vi "String value arrange_0.vi"() -> ()   [LabVIEW 2015]
panel:
  in  "Tab Control":enum32{"Page 1"}(tab)
  out "String mixx":string="100,101,102,103,104,105,106,107,108,109"
  out "Totall String charter":i32
  out "string addres":i32[](array[numeric])
  out "correct string":string[](array[string])
  out "Totall String":i16
  out "after substring":string
  out "before substring":string
  # "String value arrange"
  # "Pardeep Kumar"
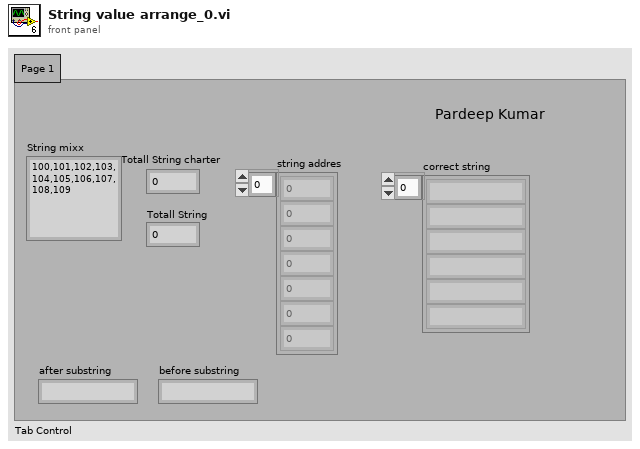
[diagram p1: front panel]
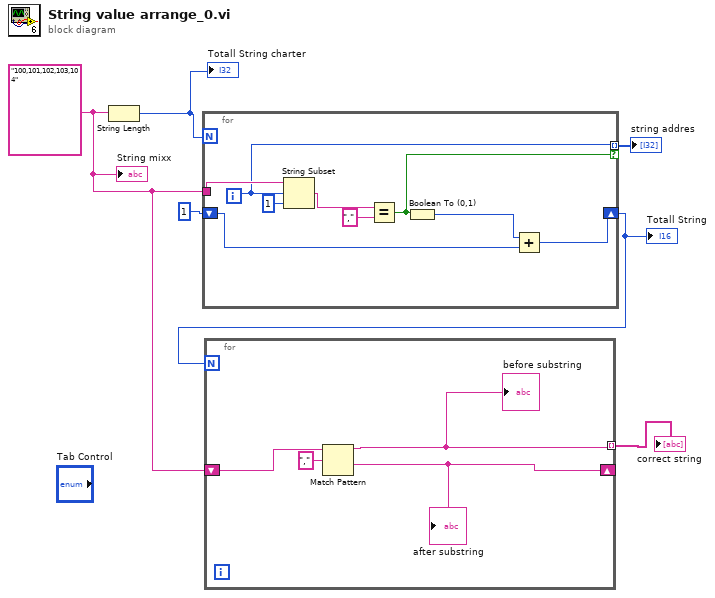
[diagram p0: block diagram]
diagram:
  w3 = "100,101,102,103,104"
  n1 = String Length(string=w3) -> (length=w6:i32)
  "Totall String charter" <- w6
  n2 = for {
    N: w6 -> [_]
    tunnel: w3 -> [w15]
    shift-right: [w10] -> w4
    shift-left: i16 1 -> [w9]
    tunnel: [w8] -> w1 mode=indexing if=w7
    i -> [w8]
    n3 = String Subset(string=w15, offset (0)=w8, length (rest)=1 ("length (rest)")) -> (substring=w13:string)
    n4 = Equal?(x=w13, y=",") -> (x = y?=w7:bool)
    n5 = Boolean To (0,1)(Boolean=w7) -> (0, 1=w11:i16)
    n6 = Add(x=w11, y=w9) -> (x+y=w10:i16)
  }
  "string addres" <- w1
  "Totall String" <- w4
  n7 = for {
    N: w4 -> [_]
    shift-right: [w16] -> _
    shift-left: w3 -> [w19]
    tunnel: [w17] -> w2 mode=indexing
    n8 = Match Pattern(string=w19, regular expression=",") -> (before substring=w17:string, after substring=w16:string)  [unwired: 1 in, 2 out]
    "after substring" <- w16
    "before substring" <- w17
  }
  "correct string" <- w2
  "String mixx" <- w3
